vi "Waveform Chart.vi"() -> ()   [LabVIEW 2023]
panel:
  in  "stop":bool
  out "Waveform Chart":dbl[](graph)
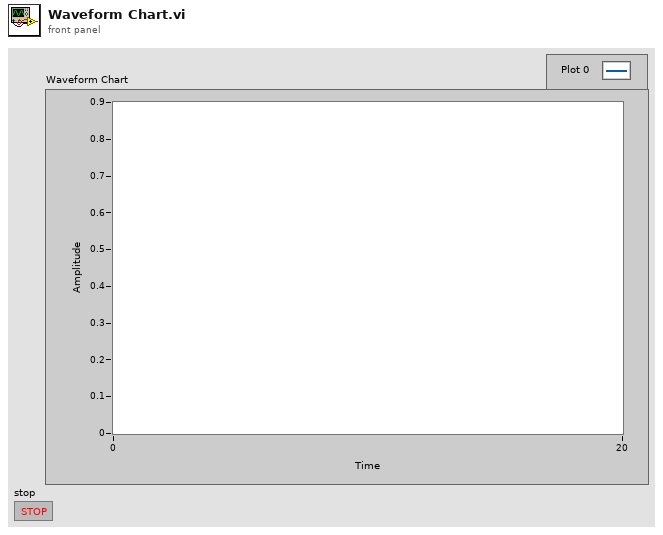
[diagram p1: front panel]
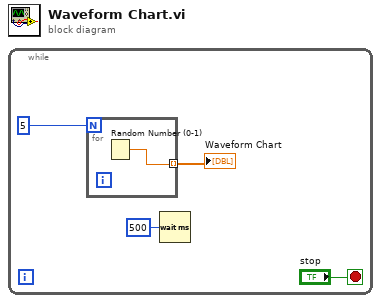
[diagram p0: block diagram]
diagram:
  n1 = while {
    stop <- "stop" stop-if-true
    n2 = for {
      N: 5 -> [_]
      tunnel: [w5] -> w1 mode=indexing
      n3 = Random Number (0-1)() -> (number: 0 to 1=w5:dbl)
    }
    "Waveform Chart" <- w1
    n4 = Wait (ms)(milliseconds to wait=u32 500) -> ()  [unwired: 1 out]
  }
